vi "GetSession.vi"(8 "error in (no error)":errorcluster, 11 "map":T1) -> (0 "error out":errorcluster, 3 "session":refnum<k21> caption="Session out")   [LabVIEW 2017, in "SystemInfoProcess.lvlib"]
uses:
  <vilib>/addons/SystemInfoProcess/SystemInfoProcess.lvlib
  <vilib>/addons/PointValueMap/controls/PointMap.ctl
  <vilib>/addons/PointValueMap/subVIs/Point_Read_variant.vi
  <vilib>/addons/PointValueMap/subVIs/Point_Write_variant.vi
  <vilib>/nisyscfg/nisyscfg.lvlib
  <vilib>/addons/PointValueMap/PointValueMap.lvlib
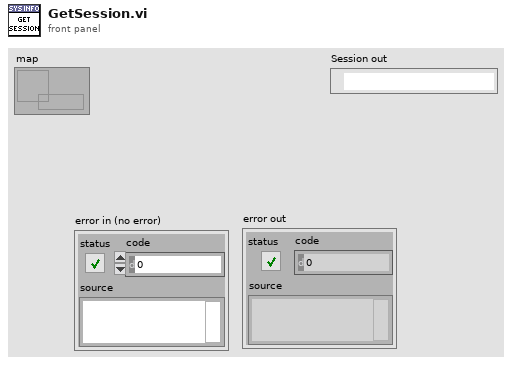
[diagram p1: front panel]
types:
  T1 = typedef "PointValueMap.lvlib/PointMap.ctl" = refnum<data-value>
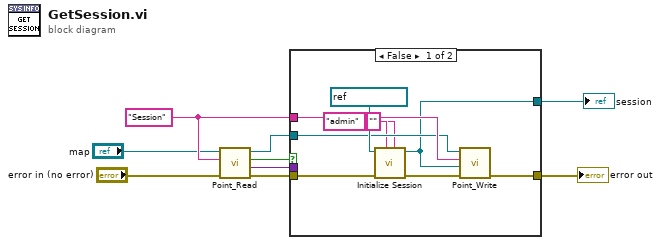
[diagram p0: block diagram]
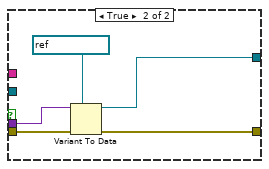
[diagram p2: hidden frame]
diagram:
  w5 = "Session" ("Tag")
  n1 = call-poly <vilib>:"Point_Read.vi"("Error In"="error in (no error)", "Tag"=w5, "Map"="map") -> ("Error Out"=w8:errorcluster, "Value"=w3:variant, "Found?"=w6:bool, "Map Out"=w7:T1)  [unwired: 3 in, 2 out]
  n2 = case shown="False" w6 {
    tunnel: w8 -> [w17 w23]
    tunnel: [w13 w22] -> w9
    tunnel: w7 -> [w14 _]
    tunnel: w5 -> [w15 _]
    tunnel: [w12 w19] -> w4
    tunnel: w3 -> [_ w20]
    frame False {
      n3 = call <vilib>:"Initialize Session.vi"("Password"="", "User Name"="admin", "error in (no error)"=w17, "Target (localhost)"=refnum<k21> "localhost" ("System Session")) -> ("error out"=w16:errorcluster, "Session out"=w12:refnum<k21>)  [unwired: 6 in]
      n4 = call-poly <vilib>:"Point_Write.vi"("Error In"=w16, "Value"=w12, "Tag"=w15, "Map"=w14) -> ("Error Out"=w13:errorcluster)  [unwired: 6 in, 1 out]
    }
    frame True {
      n5 = Variant To Data(error in=w23, type=refnum<k21> "localhost" ("System Session"), Variant=w20) -> (data=w19:refnum<k21>, error out=w22:errorcluster)
    }
  }
  "error out" <- w9
  "session" <- w4
